vi "API_Get All Inspect Data.vi"(8 "error in (no error)":errorcluster) -> (0 "error out":errorcluster, 2 "Full Inspection Data":u32[][](array[numeric]), 3 "Success":bool)   [LabVIEW 2015, in "Tool Module.lvlib"]
doc: "Retrieves all the inspection data at the end of the scan. The data is a 2D array where the rows are each a sample. Each sample has the following data:\n\nProbe Data:\n0: Sample Count HI Sample count is u16.\n1: Sample Count LO\n3: CD Error Code Error code from the collect data manager.\n4: Encoder byte 3 The encoder is 32-bits (4x U8).\n5: Encoder byte 2\n6: Encoder byte 1\n7: Encoder byte 0\n8: Tool status byte\n9: Probe Data... \n\n\nNote that the API_Get Sample Data.vi only retrieves the latest data sample. Depending on the rate it is called, significant data can be lost. At the end of the inspection use the API_Get All Inspect Data to retrieve the entire data set for processing."
uses:
  Tool Module.lvlib
  <vilib>/Utility/error.llb/Error Cluster From Error Code.vi
  <vilib>/ErrorRing/Error Ring.xnode
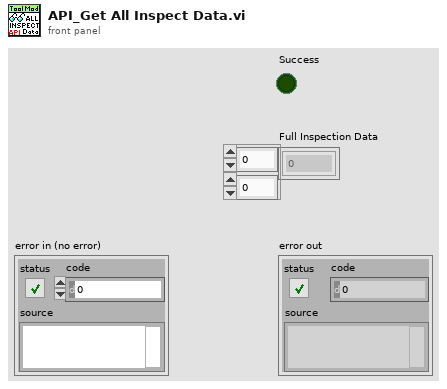
[diagram p1: front panel]
types:
  T1 = typedef "Tool Module.lvlib/Get All Inspect Data (Reply Payload)--cluster.ctl" = cluster{"Success":bool, "Full Inspection Data":u32[][]}
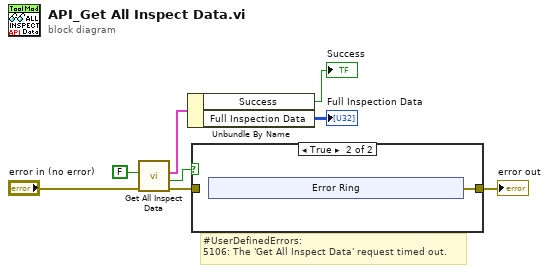
[diagram p0: block diagram]
diagram:
  # "#UserDefinedErrors:\n5106: The 'Get All Inspect Data' request timed out."
  n1 = call "Get All Inspect Data.vi"("error in (no error)"="error in (no error)", "dummy"=FALSE) -> ("error out"=w4:errorcluster, "timed out?"=w6:bool, "Reply Payload"=w3:T1)  [unwired: 7 in]
  n2 = Unbundle By Name(w3) -> ("Success"=→"Success":bool, "Full Inspection Data"=→"Full Inspection Data":u32[][])
  n3 = case shown="True" w6 {
    tunnel: [w9 w10] -> w5
    tunnel: w4 -> [w9 _]
    frame False {
    }
    frame True {
      n4 = xnode "Error Ring"() -> ("error out"=w10:errorcluster)
    }
  }
  "error out" <- w5
